vi "ReadVoltage.vi"(8 "Error In":errorcluster, 11 "reference in":refnum<class "VdAnalogInput_DAQmx.lvclass">) -> (0 "Error Out":errorcluster, 2 "Voltage":dbl, 3 "reference out":refnum<class "VdAnalogInput_DAQmx.lvclass">)   [LabVIEW 2020, in "VdAnalogInput_DAQmx.lvclass"]
uses:
  VdAnalogInput_DAQmx.lvclass
  <vilib>/DAQmx/read.llb/DAQmx Read (Analog DBL 1Chan 1Samp).vi
  <vilib>/DAQmx/miscellaneous.llb/DAQmx Fill In Error Info.vi
  VdAnalogInput_DAQmx.lvclass/VdAnalogInput_DAQmx.ctl
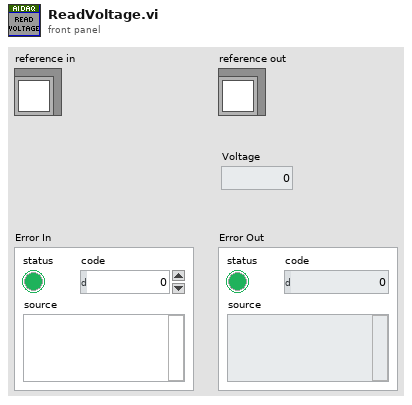
[diagram p1: front panel]
types:
  T1 = typedef "VdAnalogInput_DAQmx.lvclass/ObjectAttributes.ctl" = cluster{"task":refnum<k21>}
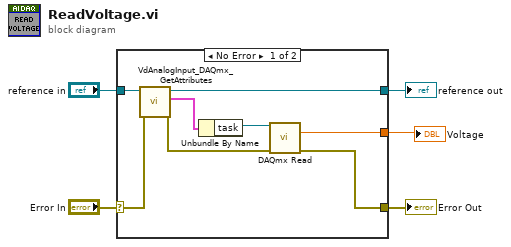
[diagram p0: block diagram]
diagram:
  n1 = case shown="No Error" "Error In" {
    selector: "Error In" -> [w13 w15]
    tunnel: [w6 w15] -> w4
    tunnel: [w10 w14] -> w2
    tunnel: "reference in" -> [w11 w14]
    tunnel: [w8 _] -> w1
    frame No Error {
      n2 = call "VdAnalogInput_DAQmx_GetAttributes.vi"("error in"=w13, "reference in"=w11) -> ("error out"=w7:errorcluster, "Data"=w12:T1, "reference out"=w10:refnum<class "VdAnalogInput_DAQmx.lvclass">)  [unwired: 6 in, 1 out]
      n3 = Unbundle By Name(w12) -> ("task"=w9:refnum<k21>)
      n4 = call-poly <vilib>:"DAQmx Read.vi"("task/channels in"=w9, "error in"=w7) -> ("data"=w8:dbl, "error out"=w6:errorcluster)  [unwired: 11 in, 1 out]
    }
    frame Error {
    }
  }
  "Error Out" <- w4
  "reference out" <- w2
  "Voltage" <- w1
